vi "Get Data.vi"(8 "error in":errorcluster, 11 "HH802U in":refnum<class "HH802U.lvclass">) -> (0 "error out":errorcluster, 2 "Data":dbl[](array[numeric]), 3 "HH802U out":refnum<class "HH802U.lvclass">)   [LabVIEW 2015, in "HH802U.lvclass"]
uses:
  HH802U.lvclass
  HH802U.lvclass/HH802U.ctl
panel:
  out "read buffer":string
  out "Datagram 2":string
  out "Datagram 1":string
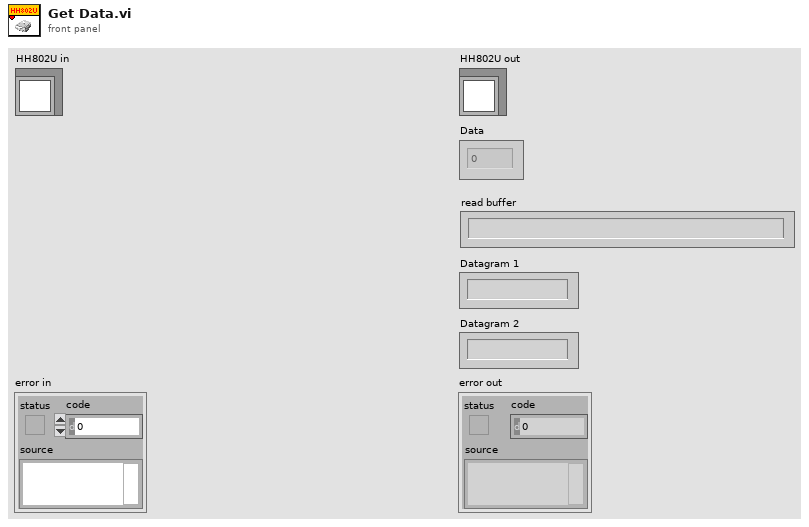
[diagram p1: front panel]
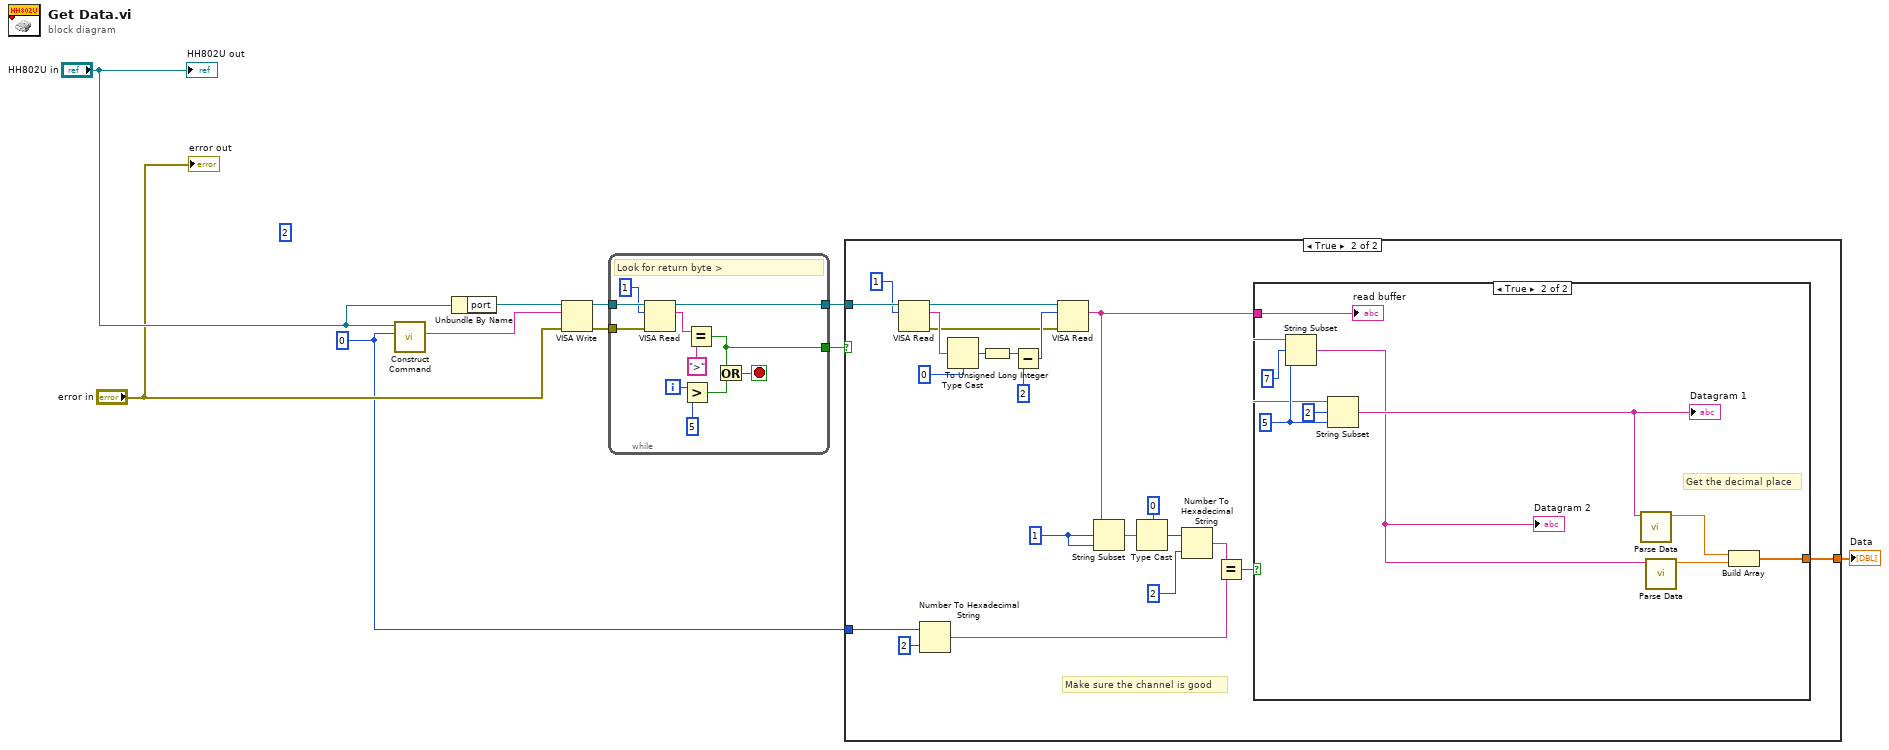
[diagram p0: block diagram]
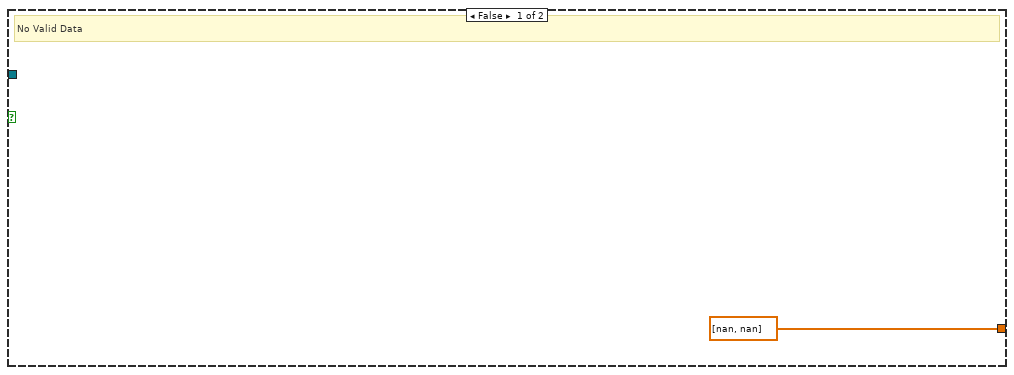
[diagram p2: hidden frame]
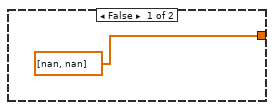
[diagram p3: hidden frame]
diagram:
  w1 = u16 0 ("Channel")
  (unwired) 2
  n1 = call "Construct Command.vi"("Channel"=w1, "HH802U in"="HH802U in") -> ("CMD"=w3:string)  [unwired: 8 in, 1 out]
  n2 = Unbundle By Name("HH802U in") -> ("port"=w2:refnum<visa-resource-name>)
  n3 = VISA Write(VISA resource name=w2, write buffer=w3, error in (no error)="error in") -> (VISA resource name out=w7:refnum<visa-resource-name>, error out=w6:errorcluster)  [unwired: 1 out]
  n4 = while {
    tunnel: w7 -> [w21]
    tunnel: w6 -> [w14]
    tunnel: [w13] -> w5
    tunnel: [w11] -> w4
    i -> [w19]
    stop <- w15 stop-if-true
    # "Look for return byte >"
    n5 = VISA Read(VISA resource name=w21, byte count=u32 1, error in (no error)=w14) -> (VISA resource name out=w13:refnum<visa-resource-name>, read buffer=w17:string)  [unwired: 2 out]
    n6 = Greater?(x=w19, y=5) -> (0:w12:bool)
    n7 = Equal?(x=w17, y=">") -> (x = y?=w11:bool)
    n8 = Or(x=w11, y=w12) -> (x .or. y?=w15:bool)
  }
  n9 = case shown="True" w4 {
    tunnel: w5 -> [_ w44]
    tunnel: [dbl[] [nan, nan] w34] -> w9
    tunnel: w1 -> [_ w29]
    frame False {
      # "No Valid Data"
    }
    frame True {
      w32 = 1 ("offset (0)")
      # "Make sure the channel is good"
      n10 = VISA Read(VISA resource name=w44, byte count=u32 1) -> (VISA resource name out=w42:refnum<visa-resource-name>, read buffer=w39:string, error out=w38:errorcluster)  [unwired: 1 in, 1 out]
      n11 = Number To Hexadecimal String(1:i16 2 ("width (-)"), 2:w29) -> (0:w24:string)
      n12 = Type Cast(type=u8 0 ("byte count"), x=w39) -> (*(type *) &x=w36:u8)
      n13 = To Unsigned Long Integer(number=w36) -> (unsigned 32bit integer=w35:u32)
      n14 = Subtract(x=w35, y=u32 2) -> (x-y=w40:u32)
      n15 = VISA Read(VISA resource name=w42, byte count=w40, error in (no error)=w38) -> (read buffer=w33:string)  [unwired: 3 out]
      n16 = String Subset(string=w33, offset (0)=w32, length (rest)=w32) -> (substring=w30:string)
      n17 = Type Cast(type=u8 0 ("byte count"), x=w30) -> (*(type *) &x=w27:u8)
      n18 = Number To Hexadecimal String(1:i16 2 ("width (-)"), 2:w27) -> (0:w25:string)
      n19 = Equal?(x=w25, y=w24) -> (x = y?=w23:bool)
      n20 = case shown="True" w23 {
        tunnel: [dbl[] [nan, nan] w46] -> w34
        tunnel: w33 -> [_ w50]
        frame False {
        }
        frame True {
          w52 = 5 ("length (rest)")
          # "Get the decimal place"
          n21 = String Subset(string=w50, offset (0)=7, length (rest)=w52) -> (substring=w49:string)
          "Datagram 2" <- w49
          n22 = String Subset(string=w50, offset (0)=2, length (rest)=w52) -> (substring=w51:string)
          "Datagram 1" <- w51
          n23 = call "Parse Data.vi"("read buffer"=w51) -> ("Numeric Control"=w47:dbl)  [unwired: 10 in]
          n24 = call "Parse Data.vi"("read buffer"=w49) -> ("Numeric Control"=w48:dbl)  [unwired: 10 in]
          n25 = Build Array(w47, w48) -> (w46:dbl[])
          "read buffer" <- w50
        }
      }
    }
  }
  "Data" <- w9
  "error out" <- "error in"
  "HH802U out" <- "HH802U in"
